vi "Database Open Connection.vi"(8 "error in":errorcluster, 11 "File Path":path) -> (0 "error out":errorcluster, 3 "valid URL":string)   [LabVIEW 2015, in "Database.lvclass"]
uses:
  Database.lvclass
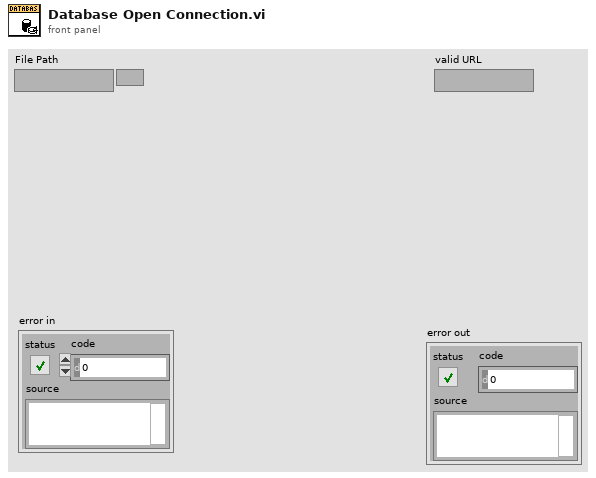
[diagram p1: front panel]
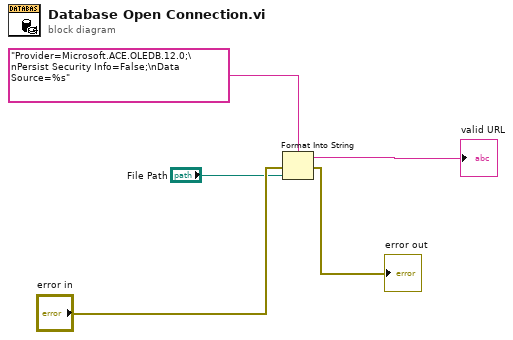
[diagram p0: block diagram]
diagram:
  n1 = Format Into String(format string="Provider=Microsoft.ACE.OLEDB.12.0;\nPersist Security Info=False;\nData Source=%s", error in="error in", "File Path") -> (resulting string=→"valid URL":string, error out=→"error out":errorcluster)  [unwired: 1 in]
